vi "Close-session.vi"(8 "error in (no error)":errorcluster, 11 "PF_MV1-D1312-240 in":refnum<class "PF_MV1-D1312-240.lvclass">) -> (0 "error out":errorcluster, 2 "IMAQ Session":refnum<k11>, 3 "PF_MV1-D1312-240 out":refnum<class "PF_MV1-D1312-240.lvclass">, 5 "Success?":bool)   [LabVIEW 2013, in "CameraVision.lvlib" / "PF_MV1-D1312-240.lvclass"]
uses:
  PF_MV1-D1312-240.lvclass
  <userlib>/Photonfocus Toolkit/_Private/Controls/pf_Camera_ctrl_mngr_action.ctl
  Camera.lvclass/Camera.ctl
  <userlib>/Photonfocus Toolkit/Photonfocus_Toolkit.lvlib
  Camera.lvclass
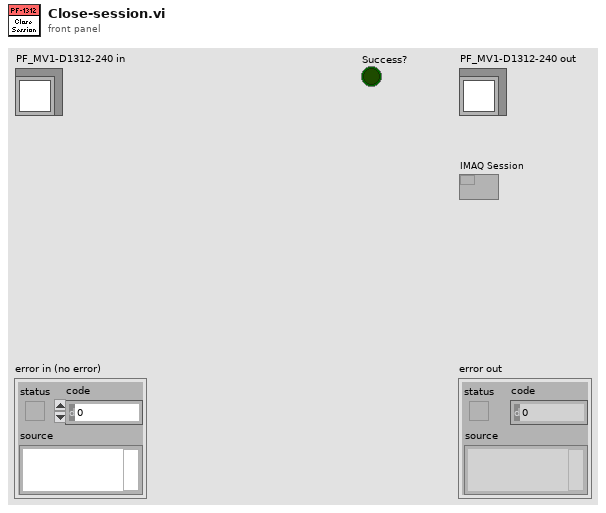
[diagram p1: front panel]
types:
  T1 = typedef "Photonfocus_Toolkit.lvlib/pf_Camera_ctrl_mngr_action.ctl" = enum16{"Create", "Destroy", "Set", "Get"}
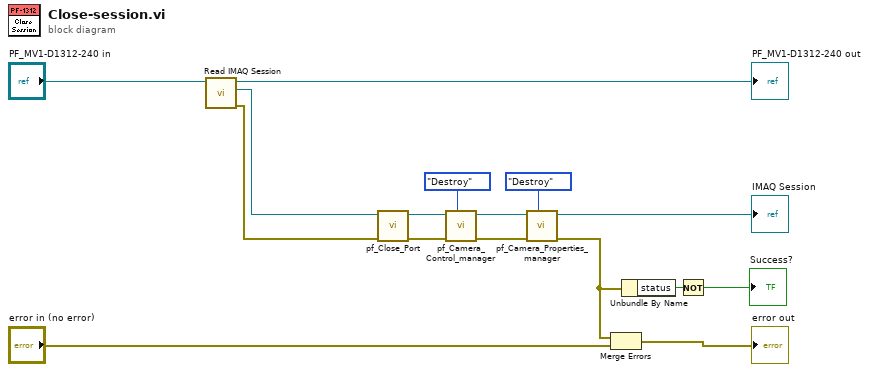
[diagram p0: block diagram]
diagram:
  n1 = call "Read IMAQ Session.vi"("Camera in"="PF_MV1-D1312-240 in") -> ("error out"=w7:errorcluster, "IMAQ Session"=w6:refnum<k11>, "Camera out"=→"PF_MV1-D1312-240 out":refnum<class "PF_MV1-D1312-240.lvclass">)  [unwired: 8 in]
  n2 = call <userlib>:"pf_Close_Port.vi"("error in (no error)"=w7, "IMAQ Session in"=w6) -> ("error out"=w8:errorcluster, "IMAQ Session out"=w13:refnum<k11>)  [unwired: 8 out]
  n3 = call <userlib>:"pf_Camera_Control_manager.vi"("Action"=pf_Camera_ctrl_mngr_action."Destroy", "error in (no error)"=w8, "IMAQ Session in"=w13) -> ("error out"=w12:errorcluster, "IMAQ Session out"=w11:refnum<k11>)  [unwired: 1 in, 6 out]
  n4 = call <userlib>:"pf_Camera_Properties_manager.vi"("Action"=pf_Camera_ctrl_mngr_action."Destroy", "error in (no error)"=w12, "IMAQ Session in"=w11) -> ("error out"=w1:errorcluster, "IMAQ Session out"=→"IMAQ Session":refnum<k11>)  [unwired: 2 in, 5 out]
  n5 = Merge Errors(w1, "error in (no error)") -> (→"error out":errorcluster)
  n6 = Unbundle By Name(w1) -> ("status"=w4:bool)
  n7 = Not(x=w4) -> (.not. x?=→"Success?":bool)
